vi "FisherPaykel Spin State.vi"(0 "VISA Refnum in":refnum<visa-resource-name>, 1 "Debug":bool, 2 "Use GEA Inverter Output":bool, 5 "Spin Profile":T3={"Target Speed (RPM)"=23, "Acceleration Rate - (10 Slowest/1000 Fastest)"=20, "Running Time (s)"=20, "Direction (CW or CCW)"=""} {"Running Time (s)" step=1; "Acceleration Rate - (10 Slowest/1000 Fastest)" min=10 max=1000 step=1; "Target Speed (RPM)" min=23 max=1600 step=1}, 7 "GEA2 Reference In":refnum<k24>, 11 "error in (no error)":errorcluster, 12 "PID":T2={"Kp"=1.84, "Ki"=0.03, "Kd"=0.0, "Kc"=0.06} {"Kc" min=0.0 max=1.0; "Kd" min=0.0 max=1.0; "Ki" min=0.0 max=1.0; "Kp" min=0.0 max=16.0}, 13 "Agitate CMD Speed":u32=150, 14 "GEA Inputs":T1={"Source"=228, "Destination"=35} {"Destination" format="%.0x"; "Source" format="%.0x"}) -> (4 "VISA Refnum out":refnum<visa-resource-name>, 8 "GEA2 Reference Out":refnum<k24>, 15 "error out":errorcluster)   [LabVIEW 2016]
uses:
  Type Definitions/Fisher Paykel Motor Profile.ctl
  Type Definitions/FisherPaykel Direction CMD.ctl
  Type Definitions/Fisher Paykel Spin PID.ctl
  Trunk/Utility/LabVIEW GEA2 Toolkit v1.0.0.0/type defs/Source_Destination.ctl
  C:/Technology Lab/NI-2010/Trunk/Utility/LabVIEW GEA2 Toolkit v1.0.0.0/Appliance.NET/GeaCommunication.dll
  Trunk/Utility/LabVIEW GEA2 Toolkit v1.0.0.0/Appliance.NET/GeaCommunication.dll
  Type Definitions/Fisher Paykel Main Command.ctl
  Trunk/Utility/LabVIEW GEA2 Toolkit v1.0.0.0/library/GEA2_Toolkit.lvlib
panel:
  out "Command (Debug) 2":string
  out "Command (Debug)":string
  # "Spin Profile Parameters"
  # "Spin Start Parameters"
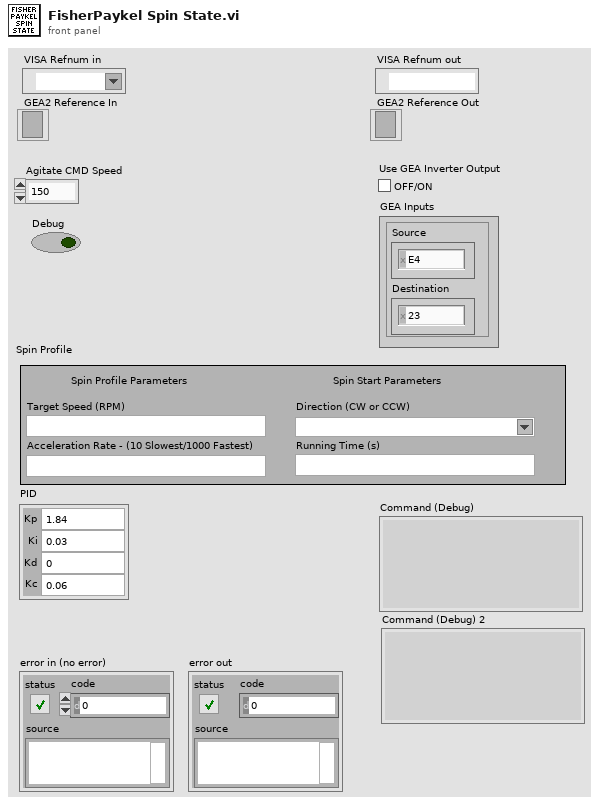
[diagram p1: front panel]
types:
  T1 = typedef "GEA2_Toolkit.lvlib/Source_Destination.ctl" = cluster{"Source":u8, "Destination":u8}
  T2 = typedef "Fisher Paykel Spin PID.ctl" = cluster{"Kp":dbl, "Ki":dbl, "Kd":dbl, "Kc":dbl}
  T3 = typedef "Fisher Paykel Motor Profile.ctl" = cluster{"Target Speed (RPM)":u16, "Acceleration Rate - (10 Slowest/1000 Fastest)":u16, "Running Time (s)":u16, "Direction (CW or CCW)":T4}
  T4 = typedef "FisherPaykel Direction CMD.ctl" = string
  T5 = typedef "Fisher Paykel Main Command.ctl" = string
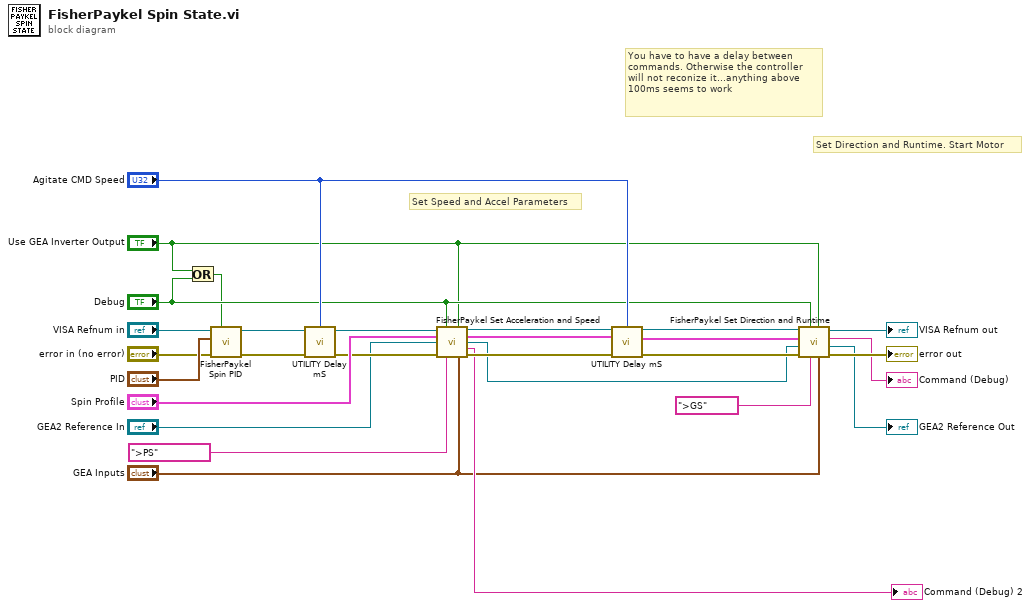
[diagram p0: block diagram]
diagram:
  # "You have to have a delay between \ncommands. Otherwise the controller\nwill not reconize it...anything above\n100ms seems to work"
  # "Set Direction and Runtime. Start Motor"
  # "Set Speed and Accel Parameters"
  n1 = Or(x="Use GEA Inverter Output", y="Debug") -> (x .or. y?=w7:bool)
  n2 = call "FisherPaykel Spin PID.vi"("Debug"=w7, "Error In"="error in (no error)", "Spin PID"="PID", "VISA Refnum in"="VISA Refnum in") -> ("Error Out"=w12:errorcluster, "VISA Refnum out"=w10:refnum<visa-resource-name>)  [unwired: 6 in]
  n3 = call "UTILITY Delay mS.vi"("Error In"=w12, "milliseconds to wait"="Agitate CMD Speed") -> ("Error Out"=w14:errorcluster)  [unwired: 13 in]
  n4 = call "FisherPaykel Set Acceleration and Speed.vi"("VISA Refnum in"=w10, "Debug"="Debug", "Use GEA Inverter Output"="Use GEA Inverter Output", "Spin Profile"="Spin Profile", "GEA2 Reference In"="GEA2 Reference In", "Error In"=w14, "Main Command"=T5 ">PS", "GEA Inputs"="GEA Inputs") -> ("VISA resource name out"=w22:refnum<visa-resource-name>, "Spin Profile Out"=w16:T3, "GEA2 Reference Out"=w3:refnum<k24>, "Command (Debug)"=→"Command (Debug) 2":string, "Error Out"=w24:errorcluster)  [unwired: 3 in]
  n5 = call "UTILITY Delay mS.vi"("Error In"=w24, "milliseconds to wait"="Agitate CMD Speed") -> ("Error Out"=w25:errorcluster)  [unwired: 13 in]
  n6 = call "FisherPaykel Set Direction and Runtime.vi"("GEA Inputs"="GEA Inputs", "Use GEA Inverter Output"="Use GEA Inverter Output", "Main Command"=T5 ">GS", "Debug"="Debug", "error in (no error)"=w25, "GEA2 Reference In"=w3, "Spin Profile"=w16, "VISA Refnum in"=w22) -> ("error out"=→"error out":errorcluster, "GEA2 Reference Out"=→"GEA2 Reference Out":refnum<k24>, "Command (Debug)"=→"Command (Debug)":string, "VISA Refnum out"=→"VISA Refnum out":refnum<visa-resource-name>)
